vi "get_config_cluster.vi"(8 "error in (no error)":errorcluster, 11 "GenericPlugin in":refnum<class "SegmenterDL100224ThreeD.lvclass">) -> (0 "error out":errorcluster, 2 "config cluster (variant)":variant, 3 "GenericPlugin out":refnum<class "SegmenterDL100224ThreeD.lvclass">)   [LabVIEW 2010, in "SegmenterDL100224ThreeD.lvclass"]
uses:
  SegmenterDL100224ThreeD.lvclass
  SegmenterDL100224ThreeD.lvclass/SegmenterDL100224ThreeD.ctl
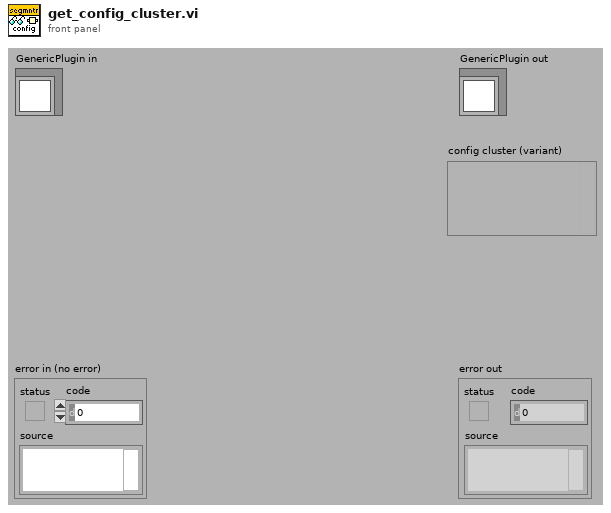
[diagram p1: front panel]
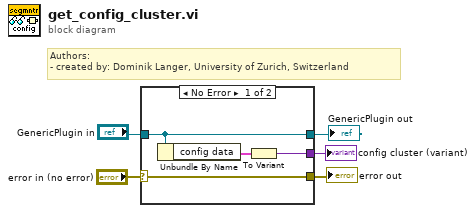
[diagram p0: block diagram]
diagram:
  # "Authors: \n- created by: Dominik Langer, University of Zurich, Switzerland"
  n1 = case shown="No Error" "error in (no error)" {
    selector: "error in (no error)" -> [w9 w10]
    tunnel: "GenericPlugin in" -> [w8 w11]
    tunnel: [w9 w10] -> w2
    tunnel: [w8 w11] -> w3
    tunnel: [w6 _] -> w1
    frame No Error {
      n2 = Unbundle By Name(w8) -> ("config data"=w7:cluster{"preprocessing macro":string})
      n3 = To Variant(anything=w7) -> (Variant=w6:variant)
    }
    frame Error {
    }
  }
  "error out" <- w2
  "GenericPlugin out" <- w3
  "config cluster (variant)" <- w1
